vi "Data_Socket.vi"() -> ()   [LabVIEW 2018]
uses:
  Global_Telescopio.vi
panel:
  out "error out 2":errorcluster
  out "error out":errorcluster
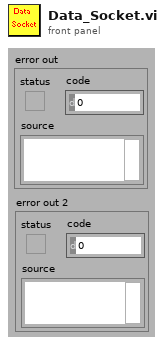
[diagram p1: front panel]
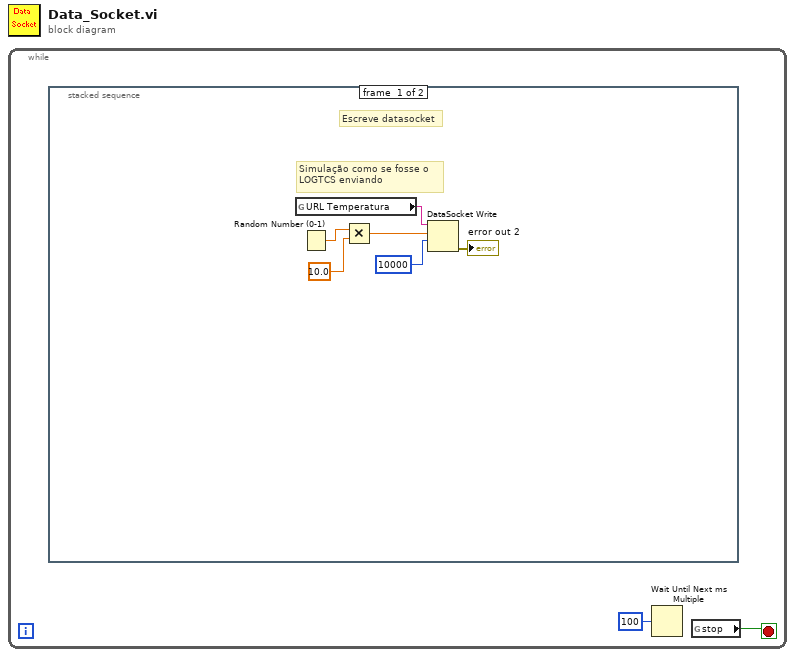
[diagram p0: block diagram]
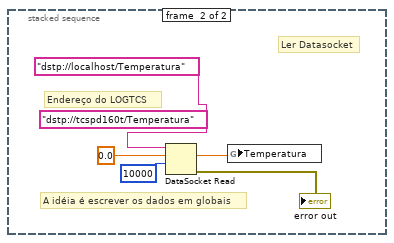
[diagram p2: hidden frame]
diagram:
  n1 = while {
    stop <- w2 stop-if-true
    n2 = stacked-sequence {
      frame #0 {
        # "Simulação como se fosse o\nLOGTCS enviando"
        # "Escreve datasocket"
        n3 = global read "Global_Telescopio.vi" "URL Temperatura"() -> (w8:string)
        n4 = Random Number (0-1)() -> (number: 0 to 1=w5:dbl)
        n5 = Multiply(x=w5, y=10.0) -> (x*y=w6:dbl)
        n6 = DataSocket Write(9:10000 ("ms timeout (0)"), 10:w6, 11:w8) -> (0:→"error out 2":errorcluster)  [unwired: 1 in, 2 out]
      }
      frame #1 {
        (unwired) "dstp://tcspd160t/Temperatura" ("URL")
        # "A idéia é escrever os dados em globais"
        # "Endereço do LOGTCS"
        # "Ler Datasocket"
        n7 = DataSocket Read(9:10000 ("ms timeout (10000)"), 10:0.0, 11:"dstp://localhost/Temperatura" ("URL")) -> (0:→"error out":errorcluster, 2:w12:dbl)  [unwired: 2 in, 5 out]
        n8 = global write "Global_Telescopio.vi" "Temperatura"(w12) -> ()
      }
    }
    n9 = Wait Until Next ms Multiple(millisecond multiple=u32 100) -> ()  [unwired: 1 out]
    n10 = global read "Global_Telescopio.vi" "stop"() -> (w2:bool)
  }
